vi "Set Log File Pretrigger Logging.vi"(8 "error in":errorcluster, 9 "pretrigger samples":i32, 10 "pretrigger logging":bool, 11 "log file in":T1 format="%.0x") -> (0 "error out":errorcluster, 3 "log file out":T1 format="%.0x")   [LabVIEW 2027, in "Embedded Data Logger Scripting.lvlib"]
uses:
  Embedded Data Logger Scripting.lvlib
  <vilib>/NI VeriStand/Custom Device API/Custom Device Item Ref.ctl
  <vilib>/NI VeriStand/Custom Device API/Set Item Property (Boolean).vi
  <vilib>/NI VeriStand/Custom Device API/Set Item Property (I32).vi
  <vilib>/NI VeriStand/Custom Device API/Custom Device API.lvlib
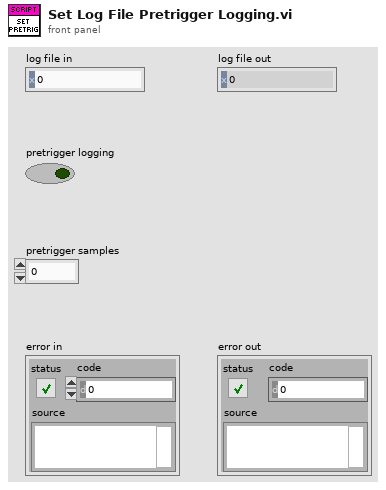
[diagram p1: front panel]
types:
  T1 = typedef "Custom Device API.lvlib/Custom Device Item Ref.ctl" = u64
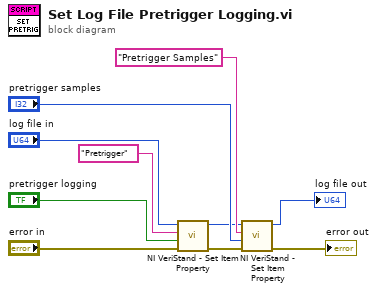
[diagram p0: block diagram]
diagram:
  n1 = call-poly <vilib>:"NI VeriStand - Set Item Property.vi"("error in (no error)"="error in", "Value"="pretrigger logging", "Property Name"="Pretrigger", "Item Ref in"="log file in") -> ("error out"=w6:errorcluster, "Item Ref out"=w4:T1)  [unwired: 6 out]
  n2 = call-poly <vilib>:"NI VeriStand - Set Item Property.vi"("error in (no error)"=w6, "Value"="pretrigger samples", "Property Name"="Pretrigger Samples", "Item Ref in"=w4) -> ("error out"=→"error out":errorcluster, "Item Ref out"=→"log file out":T1)  [unwired: 6 out]
